vi "connect.vi"(8 "error in (no error)":errorcluster, 11 "TCPClient in":refnum<class "TCPClient.lvclass">) -> (0 "error out":errorcluster, 3 "TCPClient out":refnum<class "TCPClient.lvclass">)   [LabVIEW 2016, in "TCPClient.lvclass"]
uses:
  TCPClient.lvclass
  home/plotz/lsst_ts/ss_atDome/common_labview_tcpdevice/ts_labview_tcp/TCPCommunicator/TCPCommunicator.lvclass
  TCPCommunicator/TCPCommunicator.lvclass/TCPCommunicator.ctl
  TCPSettings/TCPSettings.lvclass
  TCPCommunicator/TCPCommunicator.lvclass
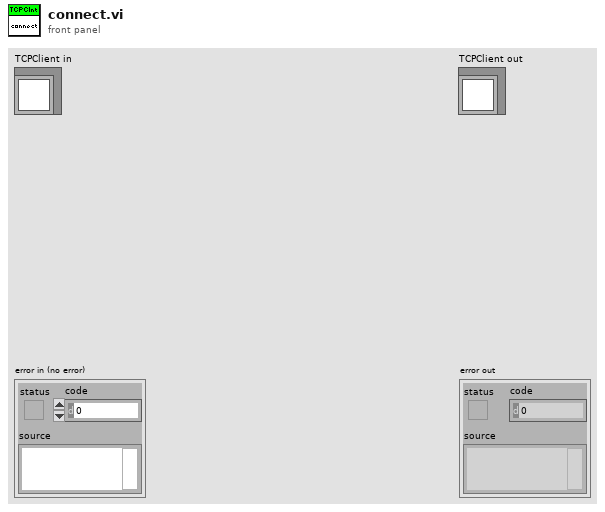
[diagram p1: front panel]
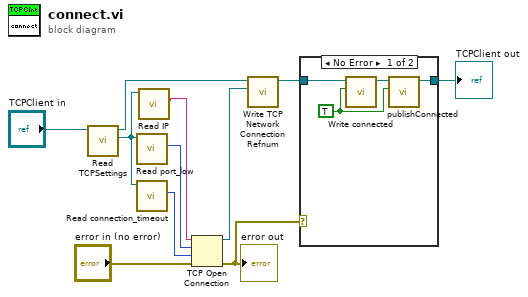
[diagram p0: block diagram]
diagram:
  n1 = call-dynamic "Read TCPSettings.vi"("TCPCommunicator in"="TCPClient in") -> ("TCPSettings.lvclass"=w2:refnum<class "TCPSettings.lvclass">, "TCPCommunicator out"=w6:refnum<class "TCPClient.lvclass">)  [unwired: 8 in, 1 out]
  n2 = call-dynamic "Read port_low.vi"("TCPSettings in"=w2) -> ("port_low"=w8:u16)  [unwired: 8 in, 2 out]
  n3 = call-dynamic "Read connection_timeout .vi"("TCPSettings in"=w2) -> ("connection_timeout"=w9:i32)  [unwired: 8 in, 2 out]
  n4 = call-dynamic "Read IP.vi"("TCPSettings in"=w2) -> ("IP"=w1:string)  [unwired: 8 in, 2 out]
  n5 = TCP Open Connection(address=w1, remote port or service name=w8, timeout ms (60000)=w9, error in (no error)="error in (no error)") -> (connection ID=w5:refnum<k5>, error out=w3:errorcluster)  [unwired: 1 in]
  "error out" <- w3
  n6 = call-dynamic "Write TCP Network Connection Refnum.vi"("TCP Network Connection Refnum"=w5, "TCPCommunicator in"=w6) -> ("TCPCommunicator out"=w7:refnum<class "TCPClient.lvclass">)  [unwired: 8 in, 1 out]
  n7 = case shown="No Error" w3 {
    tunnel: w7 -> [w15 w16]
    tunnel: [w12 w16] -> w4
    frame No Error {
      w13 = TRUE ("connected")
      n8 = call "Write connected.vi"("connected"=w13, "TCPCommunicator in"=w15) -> ("TCPCommunicator out"=w14:refnum<class "TCPClient.lvclass">)  [unwired: 8 in, 1 out]
      n9 = call-dynamic "publishConnected.vi"("Connected"=w13, "TCPCommunicator in"=w14) -> ("TCPCommunicator out"=w12:refnum<class "TCPClient.lvclass">)  [unwired: 8 in, 1 out]
    }
    frame Error {
    }
  }
  "TCPClient out" <- w4
